vi "BackgroundRunVI.vi"() -> ()   [LabVIEW 2012]
uses:
  <resource>/importtools/Common/Event/NISAST Event.lvclass
panel:
  in  "停止":bool
  out "量表":dbl(knob) scale=0.0..20.0
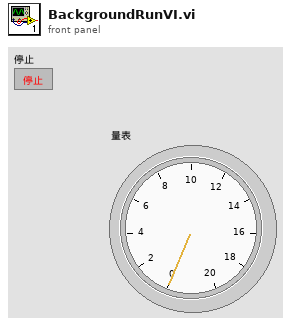
[diagram p1: front panel]
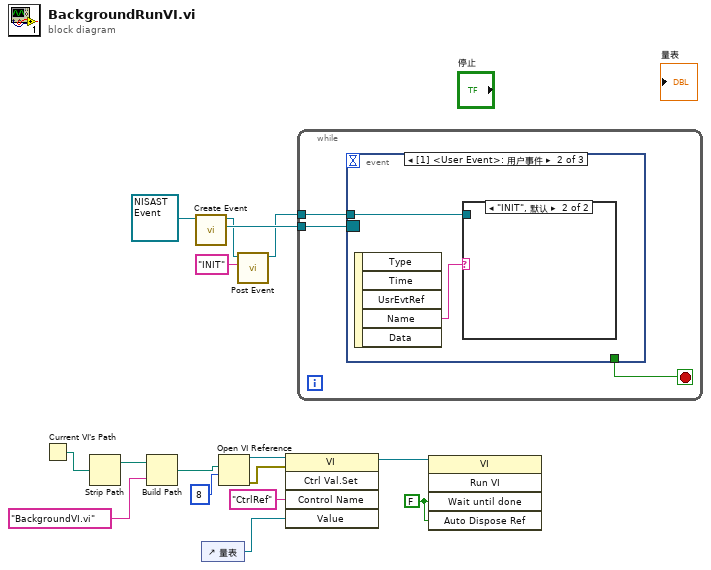
[diagram p0: block diagram]
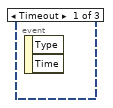
[diagram p2: hidden frame]
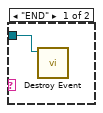
[diagram p3: hidden frame]
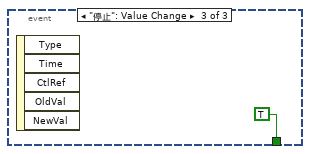
[diagram p4: hidden frame]
diagram:
  w1 = FALSE ("结束前等待")
  n1 = Current VI's Path() -> (path=w11:path)
  n2 = Strip Path(path=w11) -> (stripped path=w10:path)  [unwired: 1 out]
  n3 = Build Path(base path=w10, name or relative path="BackgroundVI.vi" ("名称或相对路径")) -> (appended path=w8:path)
  n4 = call-dynamic "Create Event.vi"("Event in"=refnum<class "NISAST Event.lvclass"> refnum ("NISAST Event.lvclass")) -> ("Event Registration Refnum"=w15:refnum<event-registration>, "Event out"=w14:refnum<class "NISAST Event.lvclass">)  [unwired: 8 in, 1 out]
  n5 = control-ref of="量表"() -> (w3:refnum<vi>)
  n6 = Open VI Reference(vi path=w8, options=8 ("选项")) -> (vi reference=w6:refnum<vi>, error out=w5:errorcluster)  [unwired: 4 in]
  n7 = call-dynamic "Post Event.vi"("Event Name"="INIT", "Event in"=w14) -> ("Event out"=w13:refnum<class "NISAST Event.lvclass">)  [unwired: 8 in, 1 out]
  n8 = invoke class="VI" method="Ctrl Val.Set"(reference=w6, error in=w5, "Control Name"="CtrlRef" ("控件名"), "Value"=w3) -> (reference out=w2:refnum<vi>)  [unwired: 1 in, 4 out]
  n9 = while {
    tunnel: w15 -> [w19]
    tunnel: w13 -> [w18]
    stop <- w17 stop-if-true
    n10 = event shown="[1] <User Event>: 用户事件" {
      selector: w19 -> [_ _ _]
      dyn-events: _ -> [_ _ _]
      timeout: _ -> [_ _ _]
      tunnel: w18 -> [_ w20 _]
      tunnel: [_ _ TRUE] -> w17
      event Timeout {
        n11 = event-data() -> ()  [unwired: 1 in, 2 out]
      }
      event User Event {
        n12 = event-data() -> ("Name"=w21:string)  [unwired: 1 in, 4 out]
        n13 = case shown="\"INIT\", 默认" w21 {
          tunnel: w20 -> [w22 _]
          frame "END" {
            n14 = call-dynamic "Destroy Event.vi"("Event in"=w22) -> ()  [unwired: 9 in, 2 out]
          }
          frame "INIT", Default {
          }
        }
      }
      event "停止": Value Change {
        n15 = event-data() -> ()  [unwired: 1 in, 5 out]
      }
    }
  }
  n16 = invoke class="VI" method="Run VI"(reference=w2, "Wait until done"=w1, "Auto Dispose Ref"=w1) -> ()  [unwired: 2 in, 5 out]
